vi "Get Current Shift Number.vi"(9 "Two Shift Pattern":bool=TRUE, 10 "refnum in":T1, 11 "Shift":string) -> (3 "Numeric":u32)   [LabVIEW 2018]
uses:
  <vilib>/Utility/config.llb/Config Data RefNum.ctl
  <vilib>/Utility/config.llb/Read Key (String).vi
  <vilib>/Utility/config.llb/NI_LVConfig.lvlib
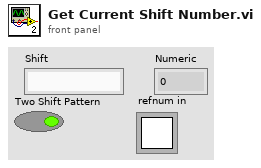
[diagram p1: front panel]
types:
  T1 = typedef "NI_LVConfig.lvlib/Config Data RefNum.ctl" = refnum<k1>
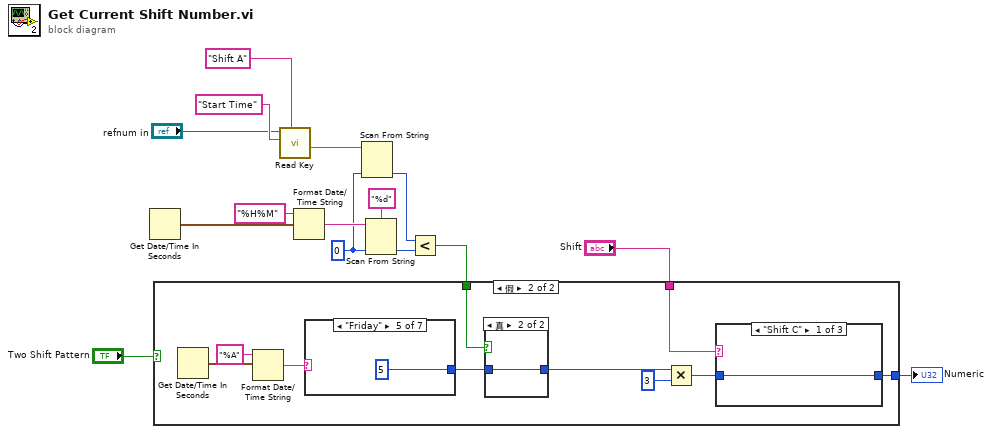
[diagram p0: block diagram]
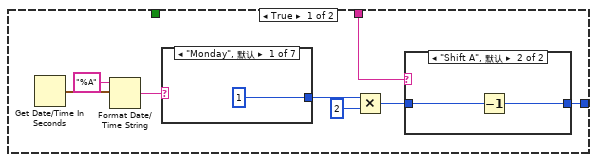
[diagram p2: hidden frame]
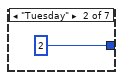
[diagram p4: hidden frame]
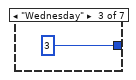
[diagram p5: hidden frame]
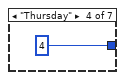
[diagram p6: hidden frame]
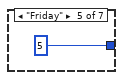
[diagram p7: hidden frame]
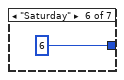
[diagram p8: hidden frame]
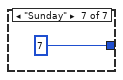
[diagram p9: hidden frame]
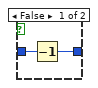
[diagram p10: hidden frame]
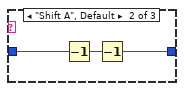
[diagram p11: hidden frame]
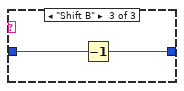
[diagram p12: hidden frame]
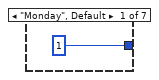
[diagram p13: hidden frame]
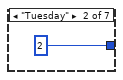
[diagram p14: hidden frame]
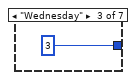
[diagram p15: hidden frame]
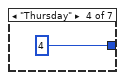
[diagram p16: hidden frame]
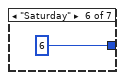
[diagram p17: hidden frame]
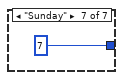
[diagram p18: hidden frame]
diagram:
  w5 = u32 0 ("default value 1")
  n1 = Get Date/Time In Seconds() -> (seconds since 1Jan1904=w9:timestamp)
  n2 = call-poly <vilib>:"Read Key.vi"("section"="Shift A", "key"="Start Time", "refnum"="refnum in") -> ("value"=w4:string)  [unwired: 5 in, 3 out]
  n3 = Format Date/Time String(time format string (%c)="%H%M", seconds (now)=w9) -> (date/time string=w11:string)  [unwired: 1 in]
  n4 = Scan From String(input string=w4, default 1=w5) -> (output 1=w3:u32)  [unwired: 3 in, 3 out]
  n5 = Scan From String(format string="%d", input string=w11, default 1=w5) -> (output 1=w2:u32)  [unwired: 2 in, 3 out]
  n6 = Less?(x=w3, y=w2) -> (x < y?=w1:bool)
  n7 = case shown="假" "Two Shift Pattern" {
    tunnel: [w23 w43] -> w15
    tunnel: "Shift" -> [w22 w42]
    tunnel: w1 -> [_ w36]
    frame True {
      n8 = Get Date/Time In Seconds() -> (seconds since 1Jan1904=w16:timestamp)
      n9 = Format Date/Time String(time format string (%c)="%A", seconds (now)=w16) -> (date/time string=w18:string)  [unwired: 1 in]
      n10 = case shown="\"Monday\", 默认" w18 {
        tunnel: [u32 1 ("Shift Number") u32 2 ("Shift Number") u32 3 ("Shift Number") u32 4 ("Shift Number") u32 5 ("Shift Number") u32 6 ("Shift Number") u32 7 ("Shift Number")] -> w21
        frame "Monday", Default {
        }
        frame "Tuesday" {
        }
        frame "Wednesday" {
        }
        frame "Thursday" {
        }
        frame "Friday" {
        }
        frame "Saturday" {
        }
        frame "Sunday" {
        }
      }
      n11 = Multiply(x=w21, y=u32 2) -> (x*y=w19:u32)
      n12 = case shown="\"Shift A\", 默认" w22 {
        tunnel: w19 -> [w24 w26]
        tunnel: [w24 w25] -> w23
        frame "Shift B" {
        }
        frame "Shift A", Default {
          n13 = Decrement(x=w26) -> (x-1=w25:u32)
        }
      }
    }
    frame False {
      n14 = Get Date/Time In Seconds() -> (seconds since 1Jan1904=w37:timestamp)
      n15 = Format Date/Time String(time format string (%c)="%A", seconds (now)=w37) -> (date/time string=w39:string)  [unwired: 1 in]
      n16 = case shown="\"Friday\"" w39 {
        tunnel: [u32 1 ("Shift Number") u32 2 ("Shift Number") u32 3 ("Shift Number") u32 4 ("Shift Number") u32 5 ("Shift Number") u32 6 ("Shift Number") u32 7 ("Shift Number")] -> w35
        frame "Monday", Default {
        }
        frame "Tuesday" {
        }
        frame "Wednesday" {
        }
        frame "Thursday" {
        }
        frame "Friday" {
        }
        frame "Saturday" {
        }
        frame "Sunday" {
        }
      }
      n17 = case shown="真" w36 {
        tunnel: w35 -> [w45 w46]
        tunnel: [w44 w46] -> w34
        frame False {
          n18 = Decrement(x=w45) -> (x-1=w44:u32)
        }
        frame True {
        }
      }
      n19 = Multiply(x=w34, y=u32 3) -> (x*y=w40:u32)
      n20 = case shown="\"Shift C\"" w42 {
        tunnel: w40 -> [w47 w50 w52]
        tunnel: [w47 w48 w51] -> w43
        frame "Shift C" {
        }
        frame "Shift A", Default {
          n21 = Decrement(x=w50) -> (x-1=w49:u32)
          n22 = Decrement(x=w49) -> (x-1=w48:u32)
        }
        frame "Shift B" {
          n23 = Decrement(x=w52) -> (x-1=w51:u32)
        }
      }
    }
  }
  "Numeric" <- w15
